vi "Detect Edge.vi"(0 "Rock":bool[][](array[boolean]), 1 "Edge F:Left | T:Right (F)":bool) -> (2 "Edge Detected ?":bool, 3 "Edge":i32)   [LabVIEW 2020, in "AoC 2022.lvlib"]
uses:
  AoC 2022.lvlib
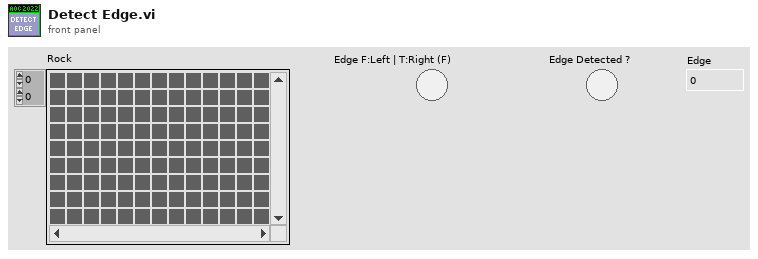
[diagram p1: front panel]
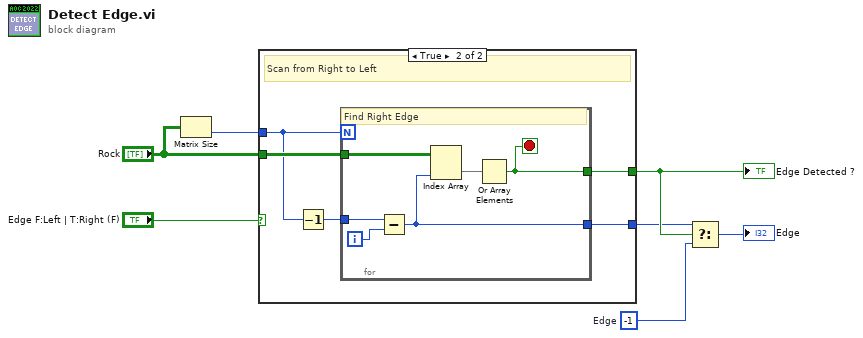
[diagram p0: block diagram]
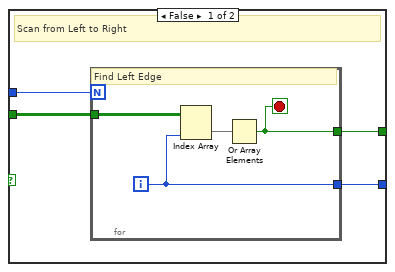
[diagram p2: hidden frame]
diagram:
  w1 = -1  # Edge
  n1 = Matrix Size(0:"Rock") -> (2:w6:i32)  [unwired: 1 out]
  n2 = case shown="True" "Edge F:Left | T:Right (F)" {
    tunnel: [w11 w20] -> w3
    tunnel: "Rock" -> [w10 w19]
    tunnel: w6 -> [w9 w17]
    tunnel: [w8 w18] -> w4
    frame False {
      # "Scan from Left to Right"
      n3 = for {
        N: w9 -> [_]
        tunnel: w10 -> [w15]
        tunnel: [w14] -> w11
        tunnel: [w12] -> w8
        i -> [w14]
        stop <- w12 stop-if-true
        # "Find Left Edge"
        n4 = Index Array(array=w15, index (col)=w14) -> (element=w13:bool[])  [unwired: 1 in]
        n5 = Or Array Elements(Boolean array=w13) -> (logical OR=w12:bool)
      }
    }
    frame True {
      # "Scan from Right to Left"
      n6 = Decrement(x=w17) -> (x-1=w16:i32)
      n7 = for {
        N: w17 -> [_]
        tunnel: w19 -> [w26]
        tunnel: [w21] -> w20
        tunnel: [w24] -> w18
        tunnel: w16 -> [w23]
        i -> [w22]
        stop <- w24 stop-if-true
        # "Find Right Edge"
        n8 = Subtract(x=w23, y=w22) -> (x-y=w21:i32)
        n9 = Index Array(array=w26, index (col)=w21) -> (element=w25:bool[])  [unwired: 1 in]
        n10 = Or Array Elements(Boolean array=w25) -> (logical OR=w24:bool)
      }
    }
  }
  "Edge Detected ?" <- w4
  n11 = Select(t=w3, s=w4, f=w1) -> (s? t:f=→"Edge":i32)
